vi "ALTS-2015 LV2GBL Work Order&Serial Number Info.vi"(7 "Options":T2=enum."Read all", 8 "error in":errorcluster, 11 "Work Order&SN Cluster In":T1) -> (0 "error out":errorcluster, 3 "Work Order&SN Cluster Out":T1)   [LabVIEW 2013]
uses:
  Controls/ALTS-2015 LV2GBL WorkOrder&SN Info Options.ctl
  Controls/ALTS-2015 WorkOrder&SN Cluster.ctl
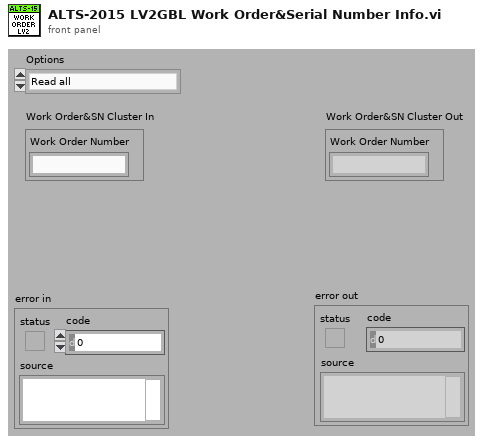
[diagram p1: front panel]
types:
  T1 = typedef "ALTS-2015 WorkOrder&SN Cluster.ctl" = cluster{"Work Order Number":string}
  T2 = typedef "ALTS-2015 LV2GBL WorkOrder&SN Info Options.ctl" = enum16{"Init", "Read all", "Write Work Order"}
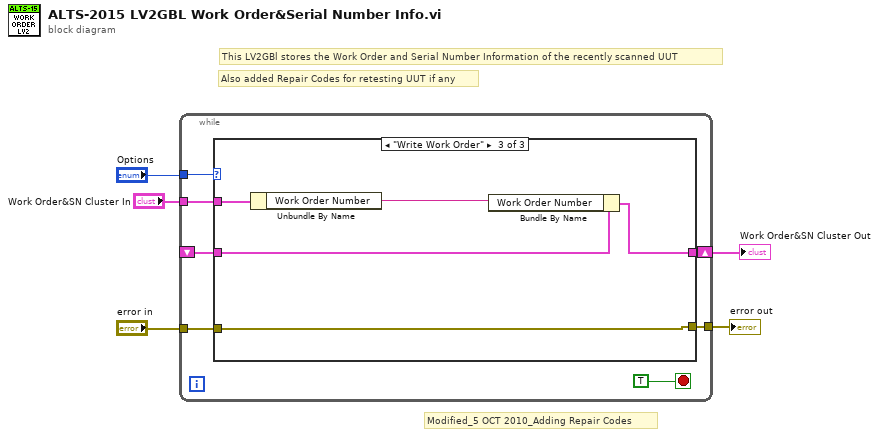
[diagram p0: block diagram]
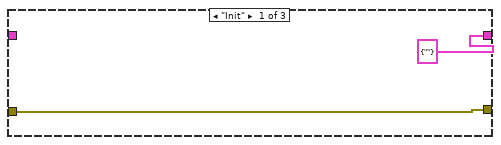
[diagram p2: hidden frame]
diagram:
  # "Also added Repair Codes for retesting UUT if any"
  # "Modified_5 OCT 2010_Adding Repair Codes"
  # "This LV2GBl stores the Work Order and Serial Number Information of the recently scanned UUT"
  n1 = while {
    tunnel: "Options" -> [w11]
    tunnel: "error in" -> [w10]
    tunnel: [w9] -> w3
    shift-right: [w7] -> w1
    shift-left: _ -> [w8]
    tunnel: "Work Order&SN Cluster In" -> [w6]
    stop <- TRUE stop-if-true
    n2 = case shown="\"Write Work Order\"" w11 {
      tunnel: [w13 w16 w21] -> w9
      tunnel: w10 -> [w13 w16 w21]
      tunnel: w8 -> [_ w15 w19]
      tunnel: [T1 {"Work Order Number"=""} ("Work Order&SN Cluster") w15 w20] -> w7
      tunnel: w6 -> [_ _ w18]
      frame "Init" {
      }
      frame "Read all", Default {
      }
      frame "Write Work Order" {
        n3 = Unbundle By Name(w18) -> ("Work Order Number"=w17:string)
        n4 = Bundle By Name(cluster=w19, "Work Order Number"=w17) -> (w20:T1)
      }
    }
  }
  "error out" <- w3
  "Work Order&SN Cluster Out" <- w1
